vi "Set Y Scale Lock.vi"(8 "error in (no error)":errorcluster, 10 "Lock":bool, 11 "Graph Manager in":refnum<class "Graph Manager.lvclass">) -> (0 "error out":errorcluster, 3 "Graph Manager out":refnum<class "Graph Manager.lvclass">)   [LabVIEW 2016, in "Graph Manager.lvclass"]
uses:
  Graph Manager.lvclass
  Graph Manager.lvclass/Graph Manager.ctl
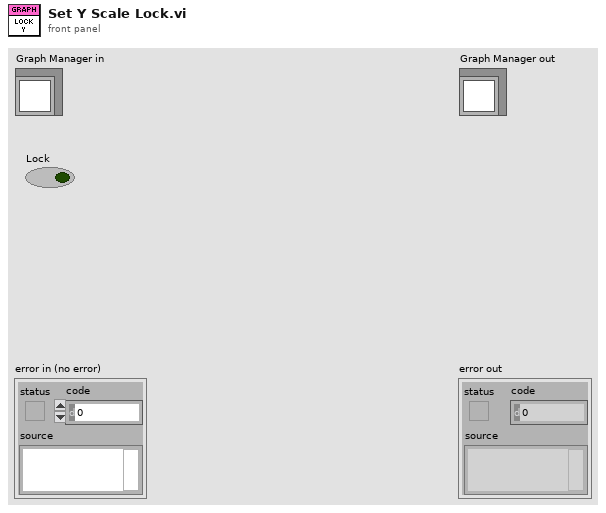
[diagram p1: front panel]
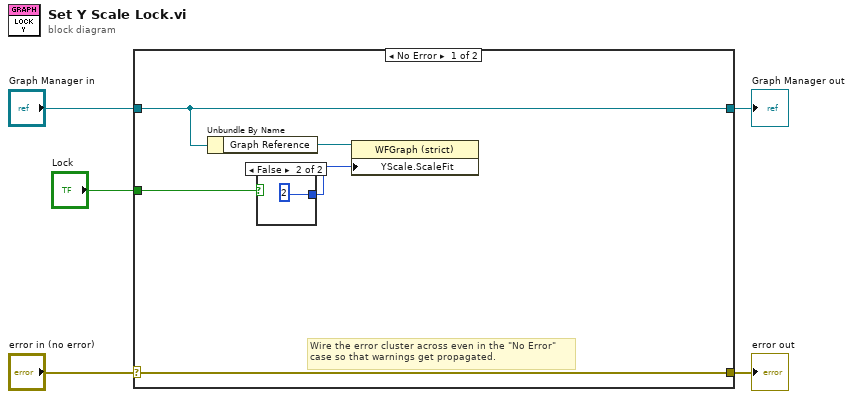
[diagram p0: block diagram]
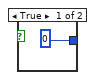
[diagram p2: hidden frame]
diagram:
  n1 = case shown="No Error" "error in (no error)" {
    selector: "error in (no error)" -> [w10 w14]
    tunnel: [w10 w14] -> w4
    tunnel: [w9 w13] -> w2
    tunnel: "Graph Manager in" -> [w9 w13]
    tunnel: "Lock" -> [w6 _]
    frame No Error {
      # "Wire the error cluster across even in the \"No Error\"\ncase so that warnings get propagated."
      n2 = Unbundle By Name(w9) -> ("Graph Reference"=w8:refnum<vi>)
      n3 = case shown="False" w6 {
        tunnel: [u8 0 ("Y Scale.Scale Fit") u8 2 ("Y Scale.Scale Fit")] -> w7
        frame True {
        }
        frame False {
        }
      }
      n4 = property class="WFGraph (strict)"(reference=w8, "YScale.ScaleFit"=w7) -> ()  [unwired: 1 in, 2 out]
    }
    frame Error {
    }
  }
  "error out" <- w4
  "Graph Manager out" <- w2
